vi "CLD 9 Step Sequencer Express Timer Front Panel.vi"() -> ()   [LabVIEW 2020]
doc: "CLD 9 Exercise"
panel:
  in  "stop 2":bool
  out "S3":dbl
  out "S2":dbl
  out "S1":dbl
  in  "Steps Selector":enum16{"Step 1", "Step 2", "Step 3"}(ring)
  out "Elapsed Time - Step 2":dbl caption="Elapsed Time (s)"
  out "Elapsed Time - Step 1":dbl caption="Elapsed Time (s)"
  out "Elapsed Time - Step 3":dbl caption="Elapsed Time (s)"
  out "Step 6":bool
  out "error IO 2":errorcluster
  in  "error IO":errorcluster
  out "Current Step time 2":dbl
  out "Elapsed Time Text":string="0  00:00:00"
  in  "Time Target (s) 3":dbl
  in  "Auto Reset 3":bool=TRUE
  in  "Reset Button 2":bool
  out "Step 5":bool
  out "Step 4":bool
  in  "stop":bool
  out "Time has Elapsed":bool
  out "Current Step Time":dbl
  out "Elapsed Time (s)":string
  out "Step 3":bool
  out "Step 2":bool
  out "Step 1":bool
  out "Time Has Elapsed":bool
  in  "Auto Reset":bool=TRUE
  in  "Reset Button":bool
  in  "Stop VI":bool
  out "error out":errorcluster
  in  "error in (no error)":errorcluster
  in  "Time Target (s)":dbl
  # "TEST1"
  # "TEST 2"
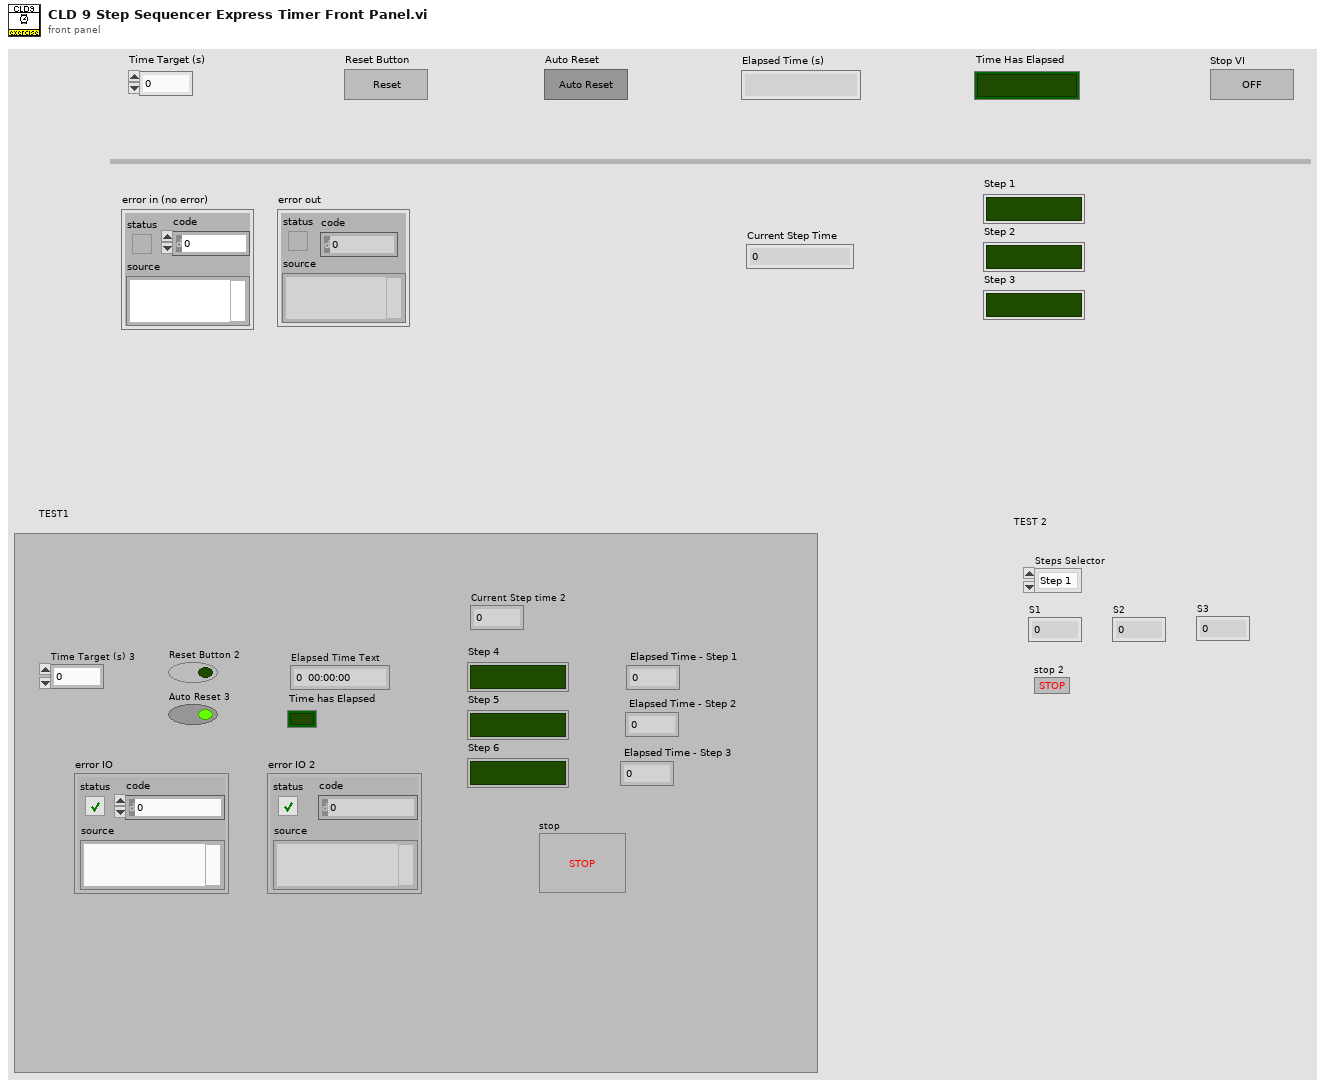
[diagram p1: front panel]
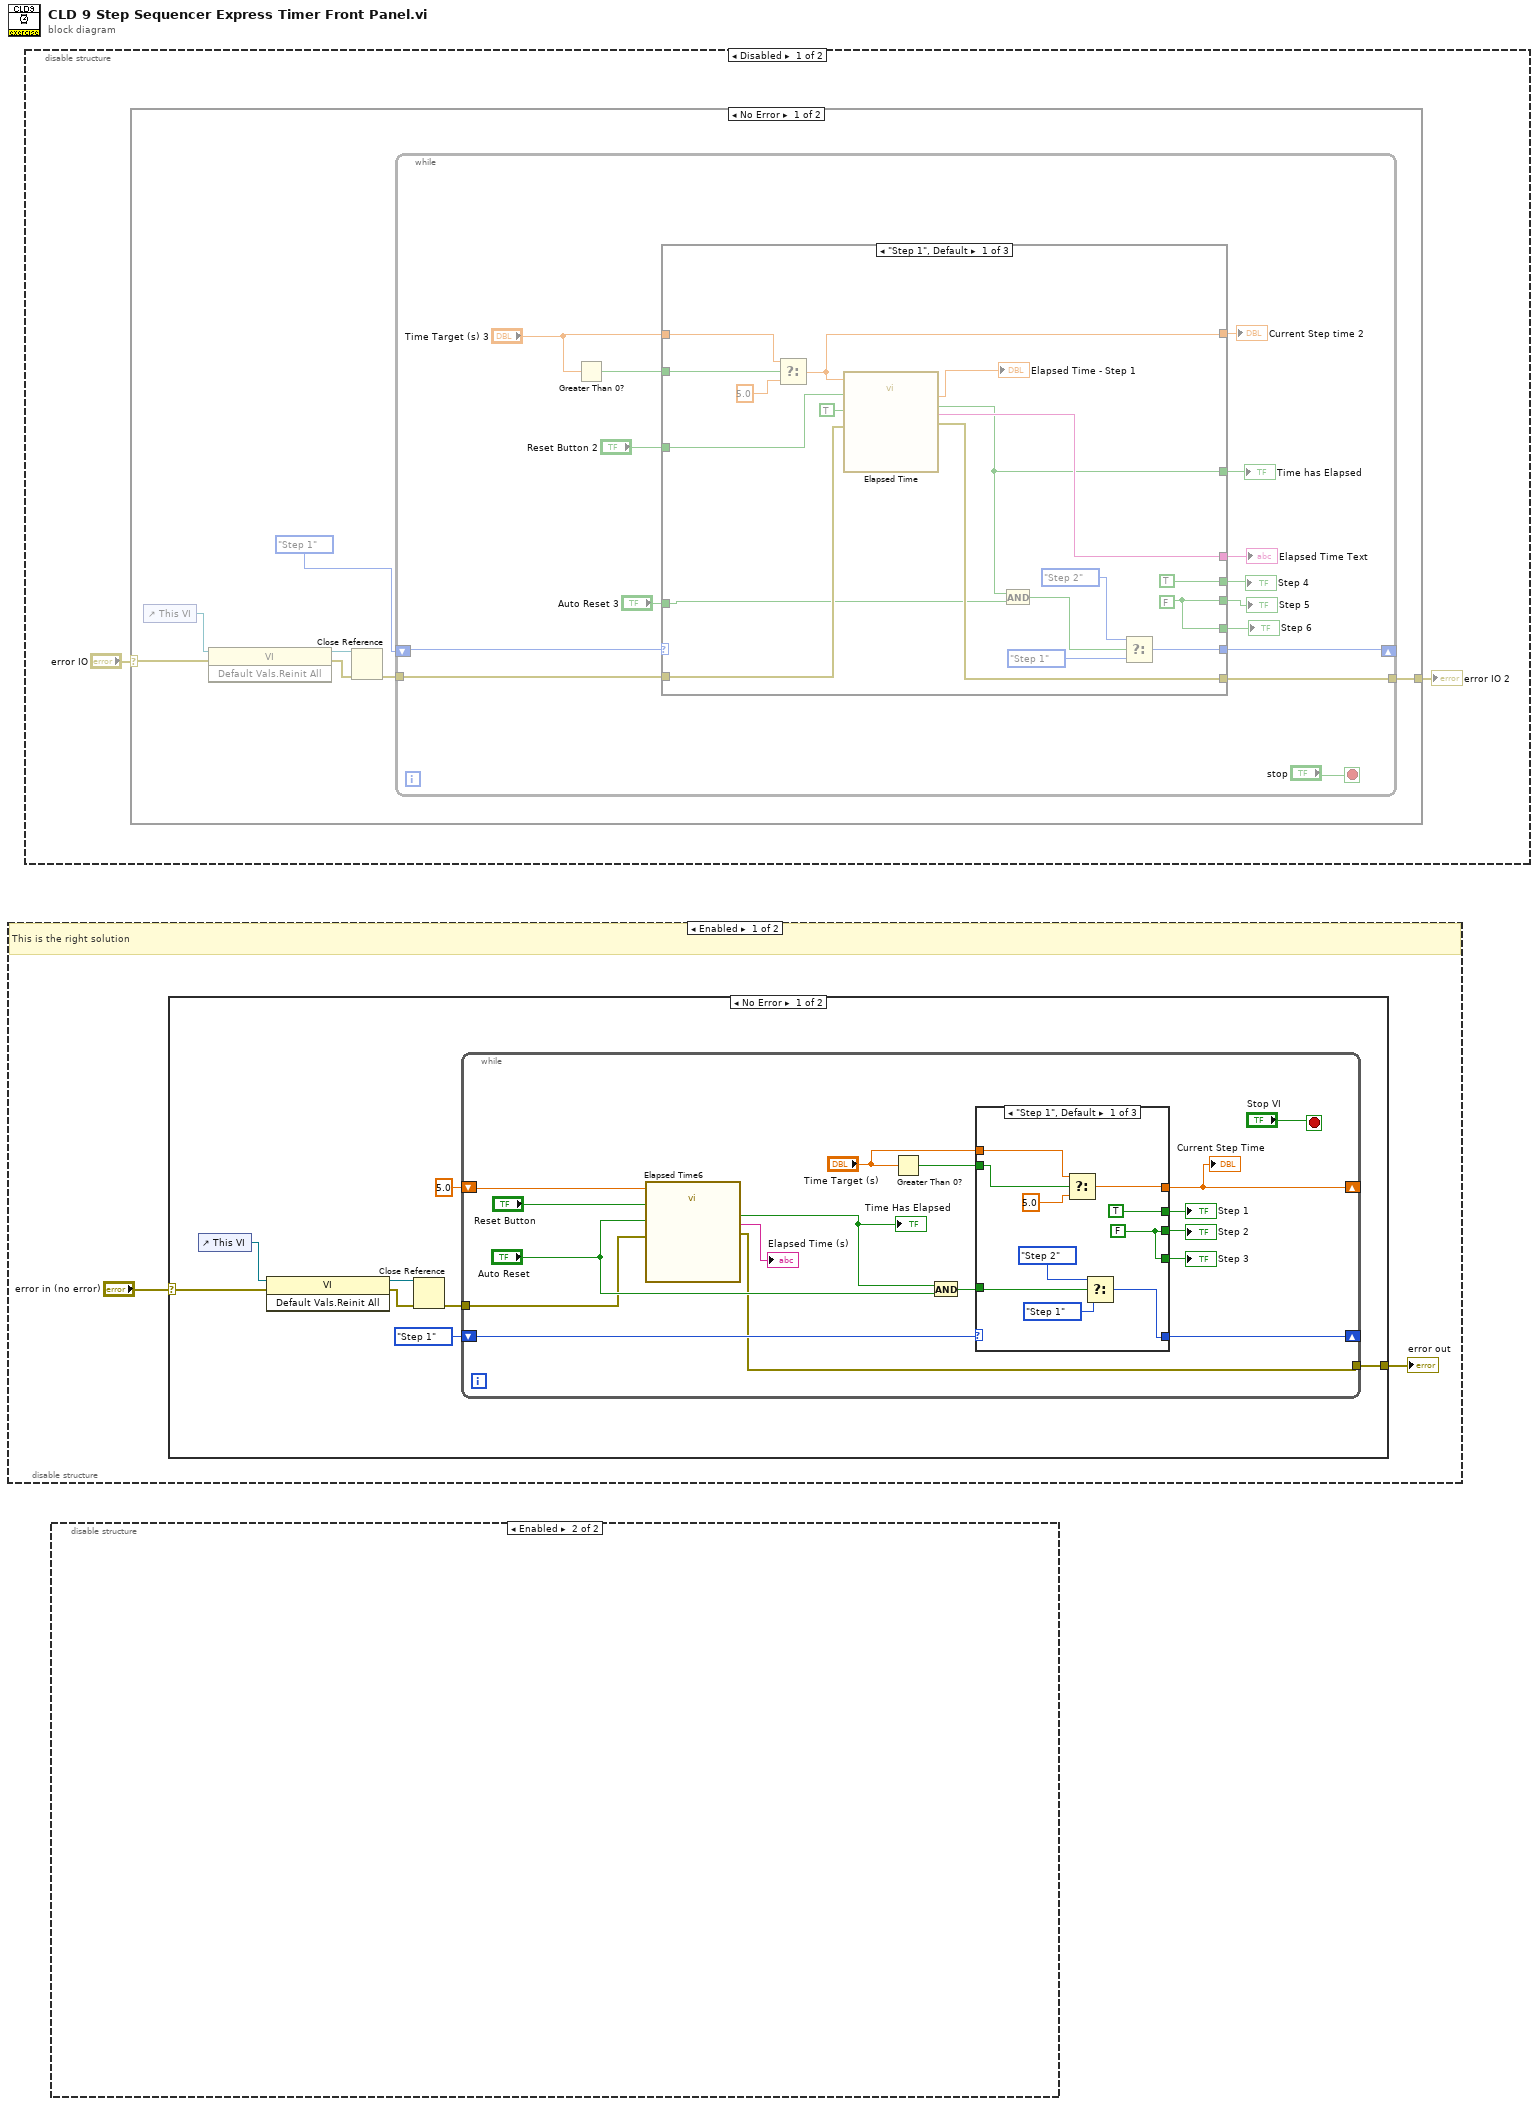
[diagram p0: block diagram]
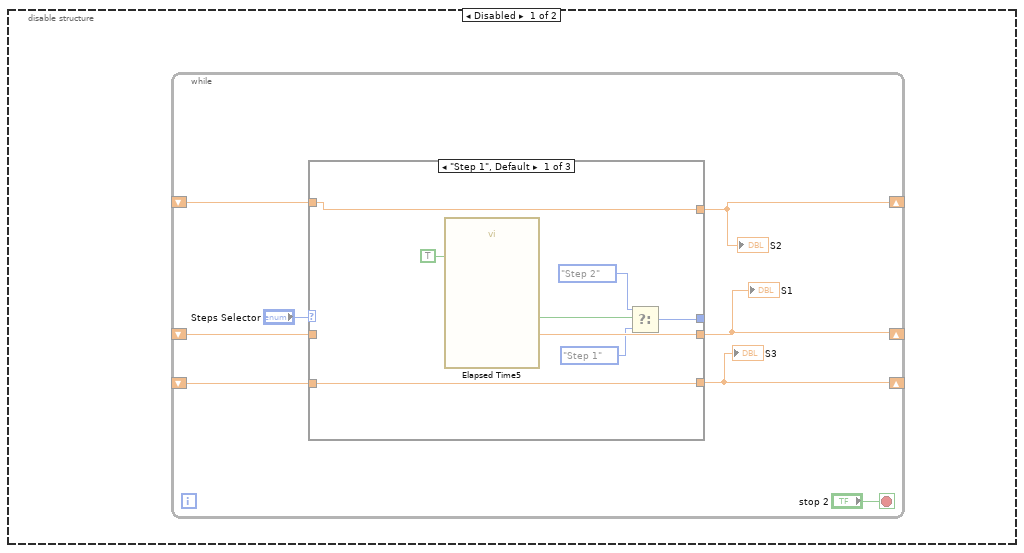
[diagram p2: hidden frame]
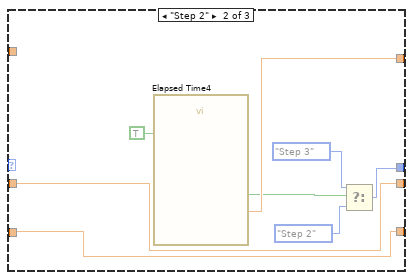
[diagram p3: hidden frame]
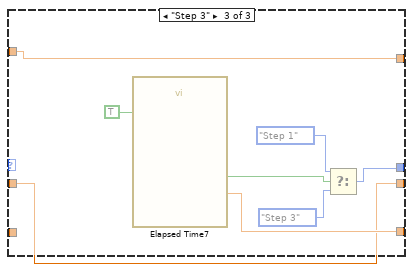
[diagram p4: hidden frame]
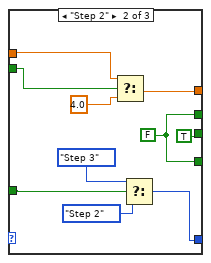
[diagram p5: hidden frame]
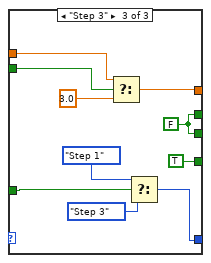
[diagram p6: hidden frame]
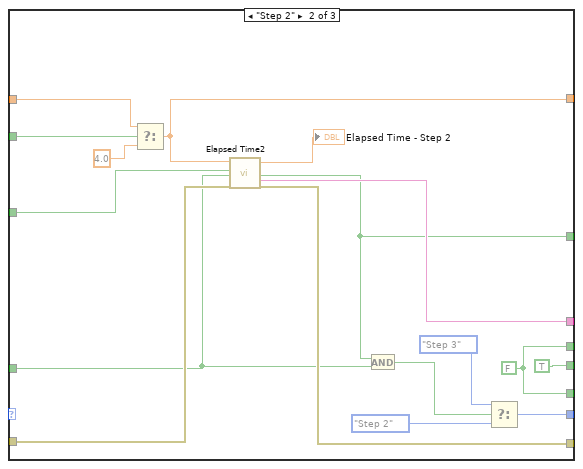
[diagram p9: hidden frame]
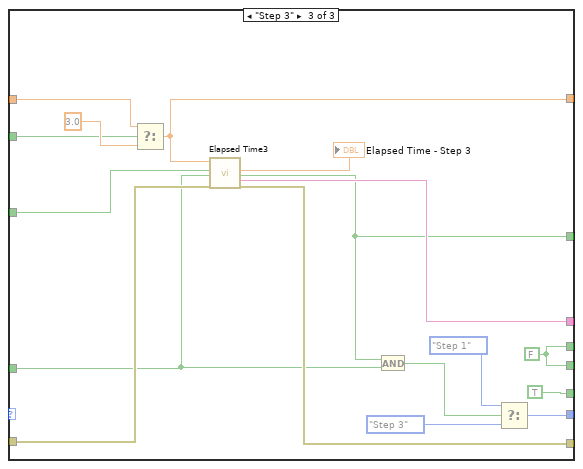
[diagram p10: hidden frame]
diagram:
  n1 = disable-structure shown="Enabled" {
    frame Enabled {
      # "This is the right solution"
      n2 = case shown="No Error" "error in (no error)" {
        selector: "error in (no error)" -> [w5 w58]
        tunnel: [w3 w58] -> w1
        frame No Error {
          n3 = control-ref of="This VI"() -> (w7:refnum<vi>)
          n4 = invoke class="VI" method="Default Vals.Reinit All"(reference=w7, error in=w5) -> (reference out=w8:refnum<vi>, error out=w6:errorcluster)  [unwired: 1 in, 1 out]
          n5 = Close Reference(reference=w8, error in (no error)=w6) -> (error out=w4:errorcluster)
          n6 = while {
            shift-right: [w26] -> _
            shift-left: enum16{"Step 1", "Step 2", "Step 3"}."Step 1" ("f") -> [w27]
            shift-right: [w12] -> _
            shift-left: 5.0 ("Time Target (s)") -> [w25]
            tunnel: w4 -> [w14]
            tunnel: [w13] -> w3
            stop <- "Stop VI" stop-if-true
            n7 = call "Elapsed Time6"("Time Target (s)"=w25, "Reset"="Reset Button", "Auto Reset"="Auto Reset", "error in (no error)"=w14) -> ("Time has Elapsed"=w11:bool, "Elapsed Time Text"=→"Elapsed Time (s)":string, "error out"=w13:errorcluster)  [unwired: 8 in, 5 out]
            "Time Has Elapsed" <- w11
            n8 = Greater Than 0?(x="Time Target (s)") -> (x > 0?=w24:bool)
            n9 = And(x=w11, y="Auto Reset") -> (x .and. y?=w23:bool)
            n10 = case shown="\"Step 1\", Default" w27 {
              tunnel: [w34 w44 w54] -> w26
              tunnel: [w30 w40 w50] -> w12
              tunnel: w23 -> [w37 w45 w55]
              tunnel: w24 -> [w32 w41 w51]
              tunnel: "Time Target (s)" -> [w31 w42 w52]
              tunnel: [TRUE ("Step 4") w38 w49] -> w18
              tunnel: [w28 TRUE ("Step 4") w49] -> w17
              tunnel: [w28 w38 TRUE ("Step 4")] -> w16
              frame "Step 1", Default {
                w28 = FALSE ("Step 4")
                n11 = Select(t=w31, s=w32, f=5.0 ("Time Target (s)")) -> (s? t:f=w30:dbl)
                n12 = Select(t=enum16{"Step 1", "Step 2", "Step 3"}."Step 2" ("f"), s=w37, f=enum16{"Step 1", "Step 2", "Step 3"}."Step 1") -> (s? t:f=w34:enum16{"Step 1", "Step 2", "Step 3"})
              }
              frame "Step 2" {
                w38 = FALSE ("Step 4")
                n13 = Select(t=w42, s=w41, f=4.0 ("Time Target (s)")) -> (s? t:f=w40:dbl)
                n14 = Select(t=enum16{"Step 1", "Step 2", "Step 3"}."Step 3" ("f"), s=w45, f=enum16{"Step 1", "Step 2", "Step 3"}."Step 2") -> (s? t:f=w44:enum16{"Step 1", "Step 2", "Step 3"})
              }
              frame "Step 3" {
                w49 = FALSE ("Step 4")
                n15 = Select(t=w52, s=w51, f=3.0 ("Time Target (s)")) -> (s? t:f=w50:dbl)
                n16 = Select(t=enum16{"Step 1", "Step 2", "Step 3"}."Step 1" ("f"), s=w55, f=enum16{"Step 1", "Step 2", "Step 3"}."Step 3") -> (s? t:f=w54:enum16{"Step 1", "Step 2", "Step 3"})
              }
            }
            "Step 1" <- w18
            "Step 3" <- w16
            "Step 2" <- w17
            "Current Step Time" <- w12
          }
        }
        frame Error {
        }
      }
      "error out" <- w1
    }
    frame Disabled {
    }
  }
  n17 = disable-structure shown="Disabled" {
    frame Disabled {
      n18 = case shown="No Error" "error IO" {
        selector: "error IO" -> [w62 w135]
        tunnel: [w66 w135] -> w59
        frame No Error {
          n19 = control-ref of="This VI"() -> (w63:refnum<vi>)
          n20 = invoke class="VI" method="Default Vals.Reinit All"(reference=w63, error in=w62) -> (reference out=w64:refnum<vi>, error out=w61:errorcluster)  [unwired: 1 in, 1 out]
          n21 = Close Reference(reference=w64, error in (no error)=w61) -> (error out=w65:errorcluster)
          n22 = while {
            shift-right: [w81] -> _
            shift-left: enum16{"Step 1", "Step 2", "Step 3"}."Step 1" ("f") -> [w70]
            tunnel: [w80] -> w66
            tunnel: w65 -> [w79]
            stop <- "stop" stop-if-true
            n23 = Greater Than 0?(x="Time Target (s) 3") -> (x > 0?=w82:bool)
            n24 = case shown="\"Step 1\", Default" w70 {
              tunnel: w82 -> [w100 w115 w132]
              tunnel: "Time Target (s) 3" -> [w99 w116 w133]
              tunnel: [w91 w107 w124] -> w81
              tunnel: [w93 w101 w123] -> w71
              tunnel: [w97 w114 w131] -> w72
              tunnel: [w96 w113 w130] -> w75
              tunnel: [TRUE ("Step 1") w111 w129] -> w74
              tunnel: [w94 TRUE ("Step 1") w129] -> w69
              tunnel: [w94 w111 TRUE ("Step 1")] -> w68
              tunnel: "Auto Reset 3" -> [w85 w104 w120]
              tunnel: "Reset Button 2" -> [w92 w103 w119]
              tunnel: w79 -> [w87 w105 w122]
              tunnel: [w86 w106 w121] -> w80
              frame "Step 1", Default {
                w94 = FALSE ("Step 1")
                n25 = Select(t=w99, s=w100, f=5.0) -> (s? t:f=w97:dbl)
                n26 = call "Elapsed Time"("Time Target (s)"=w97, "Reset"=w92, "Auto Reset"=TRUE, "error in (no error)"=w87) -> ("Elapsed Time (s)"=→"Elapsed Time - Step 1":dbl, "Time has Elapsed"=w93:bool, "Elapsed Time Text"=w96:string, "error out"=w86:errorcluster)  [unwired: 8 in, 4 out]
                n27 = And(x=w93, y=w85) -> (x .and. y?=w90:bool)
                n28 = Select(t=enum16{"Step 1", "Step 2", "Step 3"}."Step 2", s=w90, f=enum16{"Step 1", "Step 2", "Step 3"}."Step 1") -> (s? t:f=w91:enum16{"Step 1", "Step 2", "Step 3"})
              }
              frame "Step 2" {
                w111 = FALSE ("Step 1")
                n29 = Select(t=w116, s=w115, f=4.0) -> (s? t:f=w114:dbl)
                n30 = call "Elapsed Time2"("Time Target (s)"=w114, "Reset"=w103, "Auto Reset"=w104, "error in (no error)"=w105) -> ("Elapsed Time (s)"=→"Elapsed Time - Step 2":dbl, "Time has Elapsed"=w101:bool, "Elapsed Time Text"=w113:string, "error out"=w106:errorcluster)  [unwired: 8 in, 4 out]
                n31 = And(x=w101, y=w104) -> (x .and. y?=w110:bool)
                n32 = Select(t=enum16{"Step 1", "Step 2", "Step 3"}."Step 3", s=w110, f=enum16{"Step 1", "Step 2", "Step 3"}."Step 2") -> (s? t:f=w107:enum16{"Step 1", "Step 2", "Step 3"})
              }
              frame "Step 3" {
                w129 = FALSE ("Step 1")
                n33 = Select(t=w133, s=w132, f=3.0) -> (s? t:f=w131:dbl)
                n34 = call "Elapsed Time3"("Time Target (s)"=w131, "Reset"=w119, "Auto Reset"=w120, "error in (no error)"=w122) -> ("Elapsed Time (s)"=→"Elapsed Time - Step 3":dbl, "Time has Elapsed"=w123:bool, "Elapsed Time Text"=w130:string, "error out"=w121:errorcluster)  [unwired: 8 in, 4 out]
                n35 = And(x=w123, y=w120) -> (x .and. y?=w127:bool)
                n36 = Select(t=enum16{"Step 1", "Step 2", "Step 3"}."Step 1", s=w127, f=enum16{"Step 1", "Step 2", "Step 3"}."Step 3") -> (s? t:f=w124:enum16{"Step 1", "Step 2", "Step 3"})
              }
            }
            "Elapsed Time Text" <- w75
            "Step 4" <- w74
            "Step 5" <- w69
            "Current Step time 2" <- w72
            "Time has Elapsed" <- w71
            "Step 6" <- w68
          }
        }
        frame Error {
        }
      }
      "error IO 2" <- w59
    }
    frame Enabled {
    }
  }
  n37 = disable-structure shown="Enabled" {
    frame Disabled {
      n38 = while {
        shift-right: [w142] -> _
        shift-left: _ -> [w141]
        shift-right: [w140] -> _
        shift-left: _ -> [w139]
        shift-right: [w138] -> _
        shift-left: _ -> [w137]
        stop <- "stop 2" stop-if-true
        n39 = case shown="\"Step 1\", Default" "Steps Selector" {
          tunnel: [w150 w153 w160] -> w140
          tunnel: [w144 w158 w161] -> w142
          tunnel: [w145 w152 w166] -> w138
          tunnel: [w147 w154 w162] -> _
          tunnel: w141 -> [w144 _ w161]
          tunnel: w139 -> [_ w153 w160]
          tunnel: w137 -> [w145 w152 _]
          frame "Step 1", Default {
            n40 = call "Elapsed Time5"("Auto Reset"=TRUE) -> ("Elapsed Time (s)"=w150:dbl, "Time has Elapsed"=w149:bool)  [unwired: 11 in, 6 out]
            n41 = Select(t=enum16{"Step 1", "Step 2", "Step 3"}."Step 2" ("Steps Selector"), s=w149, f=enum16{"Step 1", "Step 2", "Step 3"}."Step 1" ("Steps Selector")) -> (s? t:f=w147:enum16{"Step 1", "Step 2", "Step 3"})
          }
          frame "Step 2" {
            n42 = call "Elapsed Time4"("Auto Reset"=TRUE) -> ("Elapsed Time (s)"=w158:dbl, "Time has Elapsed"=w155:bool)  [unwired: 11 in, 6 out]
            n43 = Select(t=enum16{"Step 1", "Step 2", "Step 3"}."Step 3" ("Steps Selector"), s=w155, f=enum16{"Step 1", "Step 2", "Step 3"}."Step 2" ("Steps Selector")) -> (s? t:f=w154:enum16{"Step 1", "Step 2", "Step 3"})
          }
          frame "Step 3" {
            n44 = call "Elapsed Time7"("Auto Reset"=TRUE) -> ("Elapsed Time (s)"=w166:dbl, "Time has Elapsed"=w163:bool)  [unwired: 11 in, 6 out]
            n45 = Select(t=enum16{"Step 1", "Step 2", "Step 3"}."Step 1" ("Steps Selector"), s=w163, f=enum16{"Step 1", "Step 2", "Step 3"}."Step 3" ("Steps Selector")) -> (s? t:f=w162:enum16{"Step 1", "Step 2", "Step 3"})
          }
        }
        "S1" <- w140
        "S2" <- w142
        "S3" <- w138
      }
    }
    frame Enabled {
    }
  }
